vi "grafico.vi"() -> ()   [LabVIEW 2013]
panel:
  in  "comp dc":dbl(knob) scale=-12.0..12.0
  in  "Numeric 3":i32
  out "Numeric 2":i32
  out "Waveform Chart":dbl(graph)
  out "Numeric":dbl
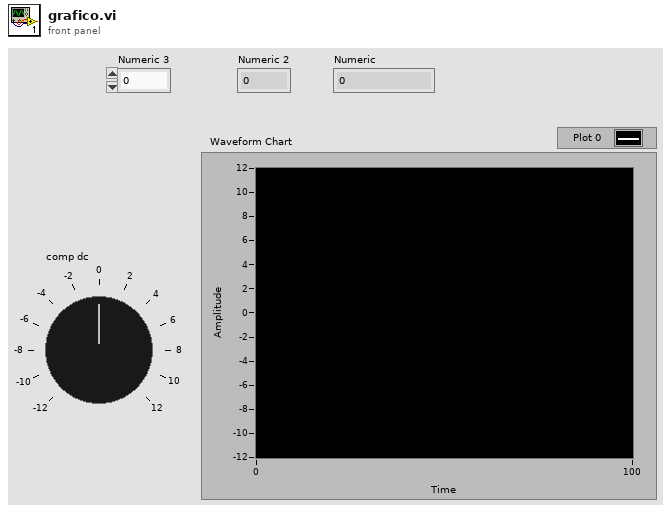
[diagram p1: front panel]
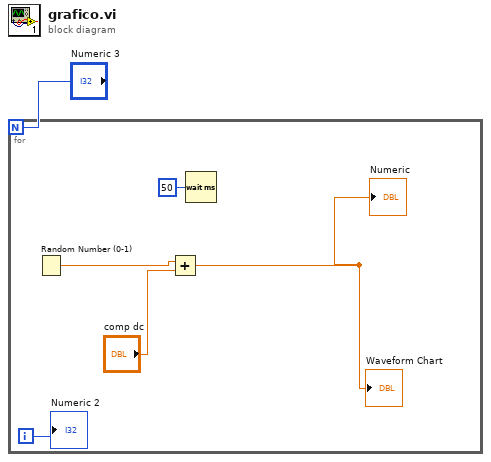
[diagram p0: block diagram]
diagram:
  n1 = for {
    N: "Numeric 3" -> [_]
    i -> [w6]
    n2 = Random Number (0-1)() -> (number: 0 to 1=w3:dbl)
    n3 = Add(x=w3, y="comp dc") -> (x+y=→"Numeric" →"Waveform Chart":dbl)
    n4 = Wait (ms)(milliseconds to wait=u32 50) -> ()  [unwired: 1 out]
    "Numeric 2" <- w6
  }
